vi "DDS Set Single-Tone Profile.vi"(0 "DDS ref in":T2={"NI USB-8451 device reference"="", "DIO port"=0, "Serial Clock Rate [kHz]"=1000}, 1 "Amplitude [dBm] (0)":dbl, 2 "Phase Offset [rad] (0)":dbl, 3 "Frequency [MHz] (0)":dbl, 5 "Channel Parameters":T1, 7 "Profile (0)":u8, 11 "error in (no error)":errorcluster, 12 "channel number (1)":u8=1 min=1 max=4 step=1) -> (4 "DDS ref out":T2={"NI USB-8451 device reference"="", "DIO port"=0, "Serial Clock Rate [kHz]"=1000}, 6 "Write Data":u8[](array[numeric]), 15 "error out":errorcluster)   [LabVIEW 2013]
doc: "Sets the amplitude/phase/frequency of the given single-tone profile on the specified channel.\n\nThe amplitude is given in units of dBm and is converted to a 14-bit amplitude scale factor using the channel's full scale output power as a parameter. The phase is given in radians and is converted to a 16-bit phase offset word. The frequency is given in MHz and is converted to a 32-bit frequency tuning word using the channel's reference clock rate as a parameter."
uses:
  DDS_box_device_reference.ctl
  <vilib>/ni845x/ni845x.llb/ni845xControl.ctl
  AD9910 registers.ctl
panel:
  out "Phase Offset Word":u32 format="%04x"
  out "Frequency Tuning Word":u32 format="%08x"
  out "Amplitude Scale Factor":u32 format="%04x"
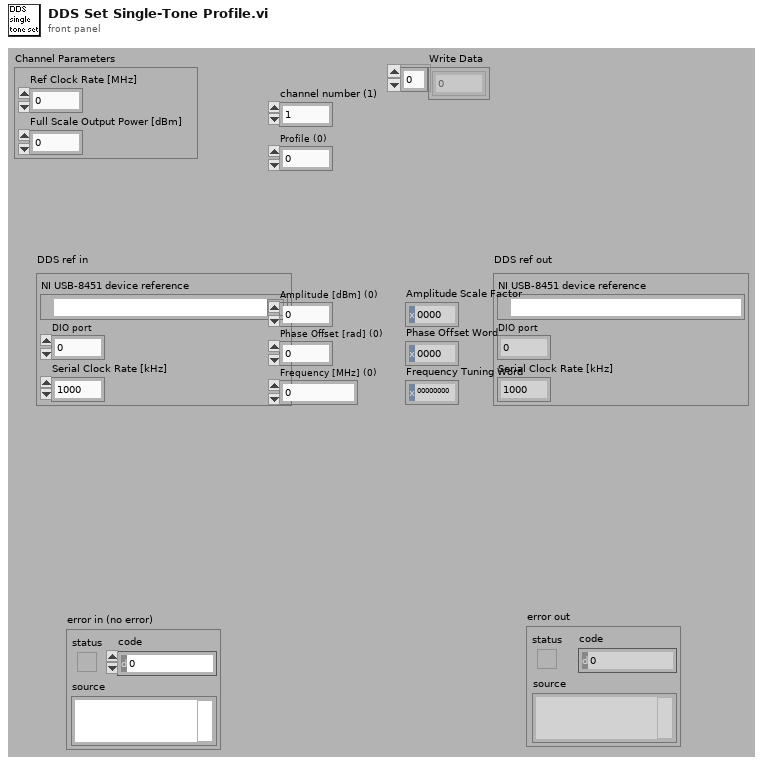
[diagram p1: front panel]
types:
  T1 = cluster{"Ref Clock Rate [MHz]":dbl, "Full Scale Output Power [dBm]":dbl}
  T2 = typedef "DDS_box_device_reference.ctl" = cluster{"NI USB-8451 device reference":T3, "DIO port":u8, "Serial Clock Rate [kHz]":u16}
  T3 = typedef "ni845xControl.ctl" = refnum<k21>
  T4 = typedef "AD9910 registers.ctl" = enum16{"CFR1", "CFR2", "CFR3", "Auxiliary DAC Control", "I/0 Update Rate", "Frequency Tuning Word", "Phase Offset Word", "Amplitude Scale Factor", "Multichip Sync", "Digital Ramp Limit", "Digital Ramp Step Size", "Digital Ramp Rate", "Single Tone Profile 0", "Single Tone Profile 1", "Single Tone Profile 2", "Single Tone Profile 3", "Single Tone Profile 4", "Single Tone Profile 5", "Single Tone Profile 6", "Single Tone Profile 7", "RAM Profile 0", "RAM Profile 1", "RAM Profile 2", "RAM Profile 3", "RAM Profile 4", "RAM Profile 5", "RAM Profile 6", "RAM Profile 7", "RAM"}
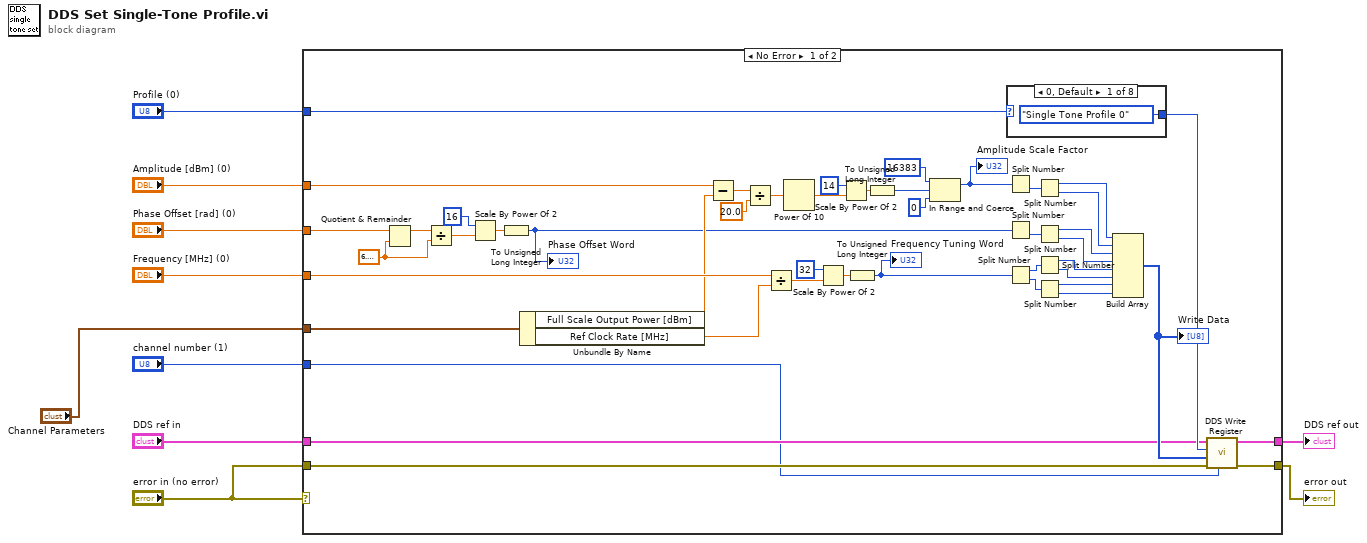
[diagram p0: block diagram]
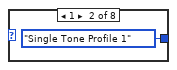
[diagram p2: hidden frame]
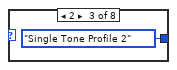
[diagram p3: hidden frame]
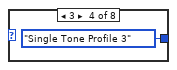
[diagram p4: hidden frame]
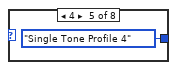
[diagram p5: hidden frame]
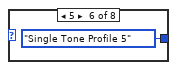
[diagram p6: hidden frame]
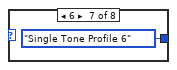
[diagram p7: hidden frame]
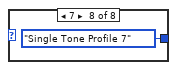
[diagram p8: hidden frame]
diagram:
  n1 = case shown="No Error" "error in (no error)" {
    tunnel: "error in (no error)" -> [w40 w66]
    tunnel: [w42 w66] -> w5
    tunnel: "Amplitude [dBm] (0)" -> [w29 _]
    tunnel: "Phase Offset [rad] (0)" -> [w18 _]
    tunnel: "Profile (0)" -> [w39 _]
    tunnel: "DDS ref in" -> [w33 w65]
    tunnel: [w41 w65] -> w4
    tunnel: "Frequency [MHz] (0)" -> [w34 _]
    tunnel: "channel number (1)" -> [w32 _]
    tunnel: "Channel Parameters" -> [w11 _]
    frame No Error {
      w12 = 6.283185307179586
      n2 = Quotient & Remainder(x=w18, y=w12) -> (x-y*floor(x/y)=w16:dbl)  [unwired: 1 out]
      n3 = Divide(x=w16, y=w12) -> (x/y=w13:dbl)
      n4 = Scale By Power Of 2(n=16, x=w13) -> (x*2^n=w15:dbl)
      n5 = To Unsigned Long Integer(number=w15) -> (unsigned 32bit integer=w14:u32)
      "Phase Offset Word" <- w14
      n6 = Unbundle By Name(w11) -> ("Full Scale Output Power [dBm]"=w30:dbl, "Ref Clock Rate [MHz]"=w31:dbl)
      n7 = Subtract(x=w29, y=w30) -> (x-y=w28:dbl)
      n8 = Divide(x=w28, y=20.0) -> (x/y=w26:dbl)
      n9 = Divide(x=w34, y=w31) -> (x/y=w36:dbl)
      n10 = Power Of 10(x=w26) -> (10^x=w25:dbl)
      n11 = Scale By Power Of 2(n=32 ("x"), x=w36) -> (x*2^n=w38:dbl)
      n12 = Scale By Power Of 2(n=14, x=w25) -> (x*2^n=w23:dbl)
      n13 = To Unsigned Long Integer(number=w38) -> (unsigned 32bit integer=w35:u32)
      "Frequency Tuning Word" <- w35
      n14 = To Unsigned Long Integer(number=w23) -> (unsigned 32bit integer=w22:u32)
      n15 = In Range and Coerce(upper limit=u32 16383, x=w22, lower limit=u32 0) -> (coerced(x)=w19:u32)  [unwired: 1 out]
      "Amplitude Scale Factor" <- w19
      n16 = Split Number(x=w19) -> (lo(x)=w53:u16)  [unwired: 1 out]
      n17 = Split Number(x=w14) -> (lo(x)=w54:u16)  [unwired: 1 out]
      n18 = Split Number(x=w35) -> (hi(x)=w55:u16, lo(x)=w56:u16)
      n19 = case shown="0, Default" w39 {
        tunnel: [AD9910_registers."Single Tone Profile 0" ("Register") AD9910_registers."Single Tone Profile 1" ("Register") AD9910_registers."Single Tone Profile 2" ("Register") AD9910_registers."Single Tone Profile 3" ("Register") AD9910_registers."Single Tone Profile 4" ("Register") AD9910_registers."Single Tone Profile 5" ("Register") AD9910_registers."Single Tone Profile 6" ("Register") AD9910_registers."Single Tone Profile 7" ("Register")] -> w43
        frame 0, Default {
        }
        frame 1 {
        }
        frame 2 {
        }
        frame 3 {
        }
        frame 4 {
        }
        frame 5 {
        }
        frame 6 {
        }
        frame 7 {
        }
      }
      n20 = Split Number(x=w53) -> (hi(x)=w45:u8, lo(x)=w46:u8)
      n21 = Split Number(x=w54) -> (hi(x)=w47:u8, lo(x)=w48:u8)
      n22 = Split Number(x=w55) -> (hi(x)=w49:u8, lo(x)=w50:u8)
      n23 = Split Number(x=w56) -> (hi(x)=w51:u8, lo(x)=w52:u8)
      n24 = Build Array(w45, w46, w47, w48, w49, w50, w51, w52) -> (w44:u8[])
      "Write Data" <- w44
      n25 = call "DDS Write Register.vi"("channel number (1)"=w32, "error in (no error)"=w40, "Write Data"=w44, "Register"=w43, "DDS ref in"=w33) -> ("error out"=w42:errorcluster, "DDS ref out"=w41:T2)  [unwired: 5 in]
    }
    frame Error {
    }
  }
  "error out" <- w5
  "DDS ref out" <- w4
